vi "tmp-camera.vi"() -> ()   [LabVIEW 2016]
uses:
  Classes/Controllers/Camera/Copy of Controller Folder/Controller.lvclass
panel:
  in  "XYZTheta":dbl[](array[numeric])=[100.0, 100.0, 0.0, 0.1]
  out "Gantry":dbl[](array[numeric])
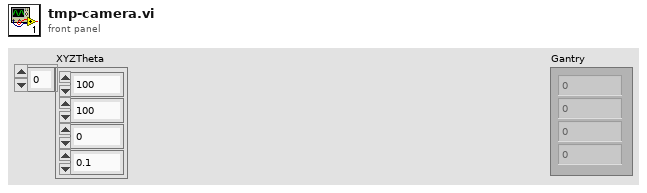
[diagram p1: front panel]
types:
  T1 = typedef "Controller.lvclass/Controllers.ctl" = cluster{"Copy of Motion.lvclass":refnum<class "Motion.lvclass">, "Copy of I-O.lvclass":refnum<class "I-O.lvclass">, "Copy of Dispenser.lvclass":refnum<class "Dispenser.lvclass">}
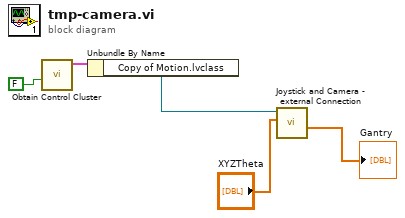
[diagram p0: block diagram]
diagram:
  n1 = call "Obtain Control Cluster.vi"("I/O"=FALSE) -> ("Control Out"=w4:T1)  [unwired: 10 in]
  n2 = Unbundle By Name(w4) -> ("Copy of Motion.lvclass"=w3:refnum<class "Motion.lvclass">)
  n3 = call "Joystick and Camera - external Connection.vi"("Motion in"=w3, "XYZTheta"="XYZTheta") -> ("Gantry"=→"Gantry":dbl[])  [unwired: 5 in, 3 out]
